vi "更新显示范围.vi"(0 "XY图输入":refnum<vi>, 1 "输出簇":T1) -> ()   [LabVIEW 2020]
uses:
  3d9fd709-47d8-4432-aed1-c192e5558cf2.vi
  2f4d84bf-9ea6-4faf-a2e7-8d22fce37656.vi
  72f31a08-3d7f-47a3-974a-597d695a0653.vi
  3c1129b5-6e40-4673-96bf-30ef819f0909.vi
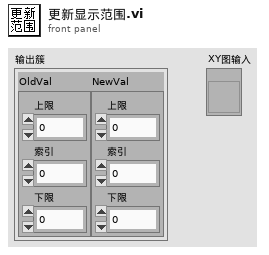
[diagram p1: front panel]
types:
  T1 = cluster{"OldVal":cluster{"上限":u32, "索引":i32, "下限":u32}, "NewVal":cluster{"上限":u32, "索引":i32, "下限":u32}}
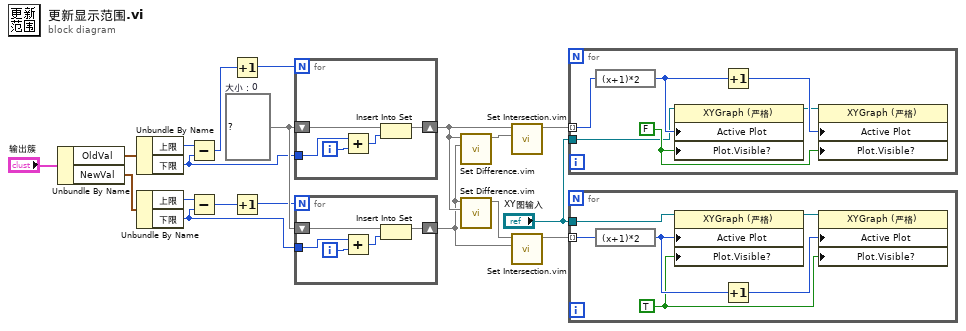
[diagram p0: block diagram]
diagram:
  w14 = set{u32} {}  # 大小：0
  n1 = Unbundle By Name("输出簇") -> ("OldVal"=w5:cluster{"上限":u32, "索引":i32, "下限":u32}, "NewVal"=w13:cluster{"上限":u32, "索引":i32, "下限":u32})
  n2 = Unbundle By Name(w5) -> ("上限"=w6:u32, "下限"=w7:u32)
  n3 = Unbundle By Name(w13) -> ("上限"=w12:u32, "下限"=w11:u32)
  n4 = Subtract(x=w6, y=w7) -> (x-y=w8:u32)
  n5 = Subtract(x=w12, y=w11) -> (x-y=w10:u32)
  n6 = Increment(x=w8) -> (x+1=w2:u32)
  n7 = Increment(x=w10) -> (x+1=w1:u32)
  n8 = for {
    N: w2 -> [_]
    tunnel: w7 -> [w24]
    shift-right: [w21] -> w18
    shift-left: w14 -> [w20]
    i -> [w23]
    n9 = Add(x=w24, y=w23) -> (x+y=w22:u32)
    n10 = Insert Into Set(10:w22, 11:w20) -> (3:w21:set{u32})  [unwired: 1 out]
  }
  n11 = for {
    N: w1 -> [_]
    tunnel: w11 -> [w29]
    shift-right: [w26] -> w17
    shift-left: w14 -> [w25]
    i -> [w28]
    n12 = Add(x=w29, y=w28) -> (x+y=w27:u32)
    n13 = Insert Into Set(10:w27, 11:w25) -> (3:w26:set{u32})  [unwired: 1 out]
  }
  n14 = call "Set Difference.vim"("set 2"=w17, "set 1"=w18) -> ("difference"=w15:set{u32})  [unwired: 9 in]
  n15 = call "Set Difference.vim"("set 2"=w18, "set 1"=w17) -> ("difference"=w19:set{u32})  [unwired: 9 in]
  n16 = call "Set Intersection.vim"("set 2"=w15, "set 1"=w18) -> ("intersection"=w9:set{u32})  [unwired: 9 in]
  n17 = call "Set Intersection.vim"("set 2"=w17, "set 1"=w19) -> ("intersection"=w16:set{u32})  [unwired: 9 in]
  n18 = for {
    tunnel: w9 -> [w35] mode=indexing
    tunnel: "XY图输入" -> [w31]
    w32 = FALSE ("曲线.可见")
    n19 = expression code="(x+1)*2"(w35) -> (w34:u32)
    n20 = property on="属性节点" class="XYGraph (严格)"(reference=w31, "Active Plot"=w34, "Plot.Visible?"=w32) -> (reference out=w30:refnum<vi>)  [unwired: 1 in, 1 out]
    n21 = Increment(x=w34) -> (x+1=w33:u32)
    n22 = property on="属性节点" class="XYGraph (严格)"(reference=w30, "Active Plot"=w33, "Plot.Visible?"=w32) -> ()  [unwired: 1 in, 2 out]
  }
  n23 = for {
    tunnel: w16 -> [w41] mode=indexing
    tunnel: "XY图输入" -> [w37]
    w38 = TRUE ("曲线.可见")
    n24 = expression code="(x+1)*2"(w41) -> (w40:u32)
    n25 = property on="属性节点" class="XYGraph (严格)"(reference=w37, "Active Plot"=w40, "Plot.Visible?"=w38) -> (reference out=w36:refnum<vi>)  [unwired: 1 in, 1 out]
    n26 = Increment(x=w40) -> (x+1=w39:u32)
    n27 = property on="属性节点" class="XYGraph (严格)"(reference=w36, "Active Plot"=w39, "Plot.Visible?"=w38) -> ()  [unwired: 1 in, 2 out]
  }
